vi "readInstructionByte.vi"(8 "error in (no error)":errorcluster, 10 "Instruction":u16, 11 "ModbusBuffer in":refnum<class "ModbusBufferBuilder.lvclass">) -> (0 "error out":errorcluster, 2 "Output":u8, 3 "ModbusBuffer out":refnum<class "ModbusBufferBuilder.lvclass">)   [LabVIEW 2016, in "ModbusBufferBuilder.lvclass"]
uses:
  ModbusBufferBuilder.lvclass
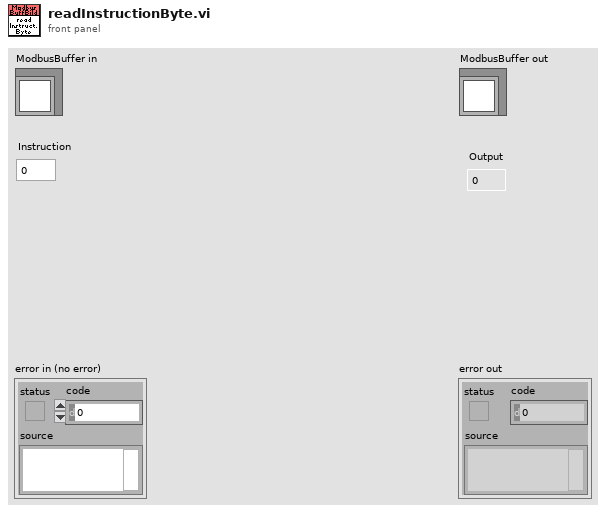
[diagram p1: front panel]
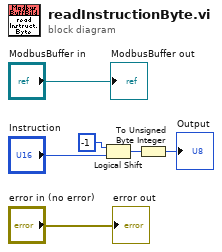
[diagram p0: block diagram]
diagram:
  n1 = Logical Shift(y=i16 -1, x="Instruction") -> (x << y=w4:u16)
  n2 = To Unsigned Byte Integer(number=w4) -> (unsigned 8bit integer=→"Output":u8)
  "error out" <- "error in (no error)"
  "ModbusBuffer out" <- "ModbusBuffer in"
